vi "Delete_Zero_Columns_Rows_Resolved_Tracks-1.vi"(4 "error IN":errorcluster, 7 "[IN] Clusters for Re\nconstructed Tracks":T1) -> (0 "error OUT":errorcluster, 3 "[OUT] Clusters for Re\nconstructed Tracks":T1)   [LabVIEW 2013]
doc: "The subVI delete zero columns and rows after resolving the problem point"
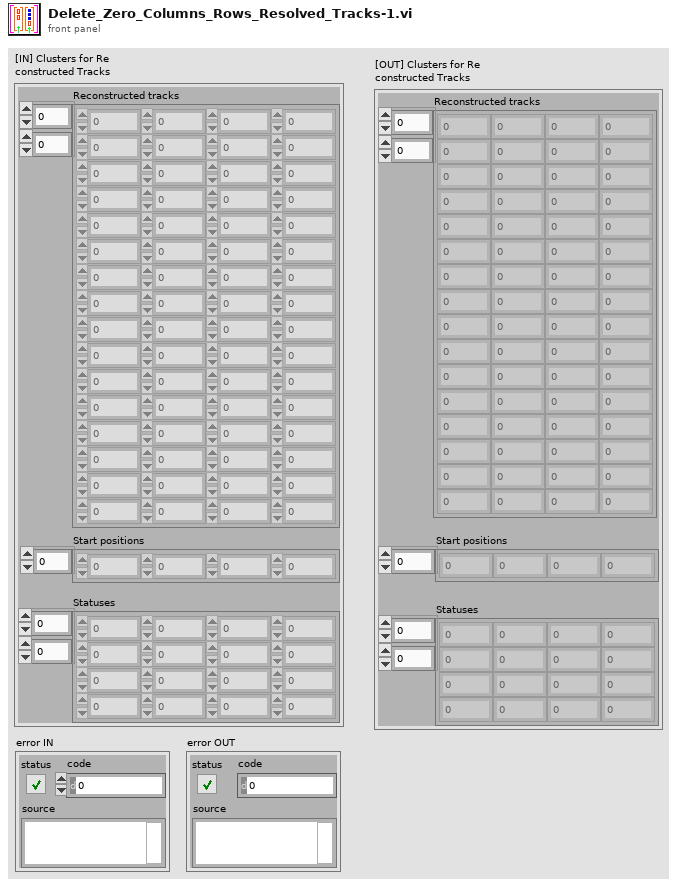
[diagram p1: front panel]
types:
  T1 = cluster{"Reconstructed tracks":dbl[][], "Start positions":i32[], "Statuses":i16[][]}
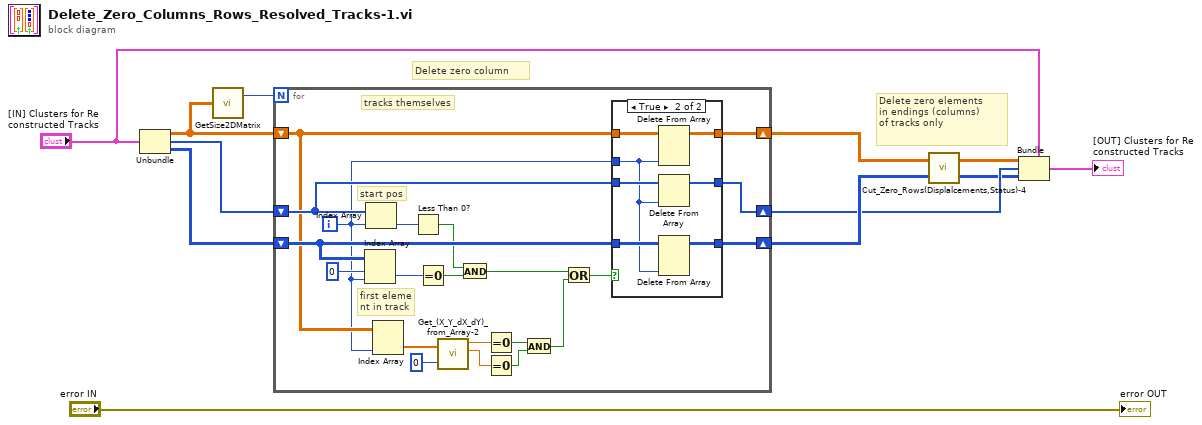
[diagram p0: block diagram]
diagram:
  # "Delete zero elements \nin endings (columns)\nof tracks only"
  # "Delete zero column"
  n1 = Unbundle("[IN] Clusters for Re\nconstructed Tracks") -> ("Reconstructed tracks"=w11:dbl[][], "Start positions"=w10:i32[], "Statuses"=w9:i16[][])
  n2 = call "GetSize2DMatrix.vi"("Array IN (2D)"=w11) -> ("# Cols"=w12:i32)  [unwired: 1 out]
  n3 = for {
    N: w12 -> [_]
    shift-right: [w28] -> w7
    shift-left: w11 -> [w22]
    shift-right: [w27] -> w5
    shift-left: w10 -> [w30]
    shift-right: [w26] -> w6
    shift-left: w9 -> [w29]
    i -> [w21]
    # "tracks themselves"
    # "start pos"
    # "first eleme\nnt in track"
    n4 = Index Array(array=w29, index (row)=0, index (col)=w21) -> (element=w31:i16)
    n5 = Index Array(array=w30, index=w21) -> (element=w32:i32)
    n6 = Index Array(array=w22, index (col)=w21) -> (element=w20:dbl[])  [unwired: 1 in]
    n7 = Less Than 0?(x=w32) -> (x < 0?=w24:bool)
    n8 = Equal To 0?(x=w31) -> (x = 0?=w25:bool)
    n9 = call "Get_(X_Y_dX_dY)_from_Array-2.vi"("(X,Y,dX,dY)"=w20, "Index of Displacement"=0) -> ("X"=w18:dbl, "Y"=w17:dbl)  [unwired: 2 out]
    n10 = And(x=w24, y=w25) -> (x .and. y?=w23:bool)
    n11 = Equal To 0?(x=w18) -> (x = 0?=w16:bool)
    n12 = Equal To 0?(x=w17) -> (x = 0?=w15:bool)
    n13 = And(x=w16, y=w15) -> (x .and. y?=w13:bool)
    n14 = Or(x=w23, y=w13) -> (x .or. y?=w14:bool)
    n15 = case shown="True" w14 {
      tunnel: w22 -> [w36 w43]
      tunnel: w21 -> [_ w37]
      tunnel: w30 -> [w35 w42]
      tunnel: w29 -> [w34 w39]
      tunnel: [w36 w41] -> w28
      tunnel: [w35 w40] -> w27
      tunnel: [w34 w38] -> w26
      frame False {
      }
      frame True {
        n16 = Delete From Array(array=w43, index (col)=w37) -> (array with subset deleted=w41:dbl[][])  [unwired: 2 in, 1 out]
        n17 = Delete From Array(array=w42, index=w37) -> (array with subset deleted=w40:i32[])  [unwired: 1 in, 1 out]
        n18 = Delete From Array(array=w39, index (col)=w37) -> (array with subset deleted=w38:i16[][])  [unwired: 2 in, 1 out]
      }
    }
  }
  n19 = call "Cut_Zero_Rows(Displalcements,Status)-4.vi"("[IN] Dot matrix\nwith zero points"=w6, "[IN] (X,Y,dX,dY) \nwith zero displ"=w7) -> ("[OUT] Dot \nMatrix"=w3:i16[][], "[OUT] (X,Y,dX,dY)\nw/t zero displac"=w4:dbl[][])
  n20 = Bundle(cluster="[IN] Clusters for Re\nconstructed Tracks", "Reconstructed tracks"=w4, "Start positions"=w5, "Statuses"=w3) -> (→"[OUT] Clusters for Re\nconstructed Tracks":T1)
  "error OUT" <- "error IN"
